vi "fastFrame_wave_to_bg_and_mol_signal.vi"(4 "all fast frames":dbl[](array[numeric])) -> (0 "ave. molecularTD signal":dbl[](array[numeric]), 1 "cor. ave. TD signal":dbl[](array[numeric]), 2 "ave. background TD signal":dbl[](array[numeric]))   [LabVIEW 2011]
doc: "This VI takes the wavform measured by the OSC and calculates the average signal for both the background as well as the molecular cylce. It also creates the substracted array (i.e. molecular - background signal)"
uses:
  global.vi
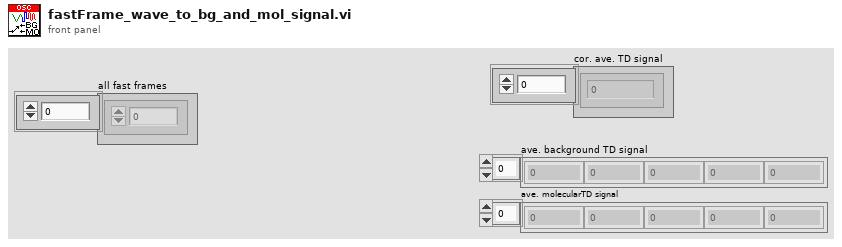
[diagram p1: front panel]
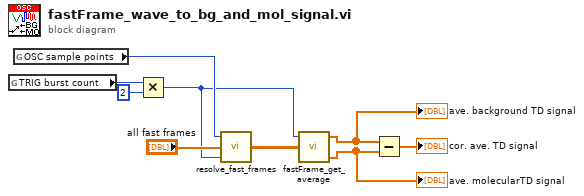
[diagram p0: block diagram]
diagram:
  n1 = global read "global.vi" "TRIG burst count"() -> (w3:i32)
  n2 = global read "global.vi" "OSC sample points"() -> (w8:i32)
  n3 = Multiply(x=w3, y=2) -> (x*y=w1:i32)
  n4 = call "resolve_fast_frames.vi"("fast frame count"=w1, "all fast frames"="all fast frames", "sample points per frame"=w8) -> ("resolved waveforms"=w7:dbl[][])  [unwired: 2 in]
  n5 = call "fastFrame_get_average.vi"("array"=w7, "fast frame count"=w1) -> ("averaged molecular frames"=w4:dbl[], "averaged background frames"=w5:dbl[])  [unwired: 2 in]
  "ave. background TD signal" <- w5
  "ave. molecularTD signal" <- w4
  n6 = Subtract(x=w5, y=w4) -> (x-y=→"cor. ave. TD signal":dbl[])
